vi "TreeFirstitem.vi"(8 "error in (no error)":errorcluster, 10 "queue in":refnum<queue>, 11 "TreeControl in":refnum<vi>) -> (0 "error out":errorcluster)   [LabVIEW 2019]
doc: "If the tree has values select the first and send the queue to show it"
uses:
  <vilib>/Bytelabs/ByteSimpleQ/ByteSimpleQ/Typedefs/message_cluster.ctl
  TypeDef/SubPanelType.ctl
  <vilib>/Bytelabs/ByteSimpleQ/ByteSimpleQ/ByteSimpleQ.lvlib
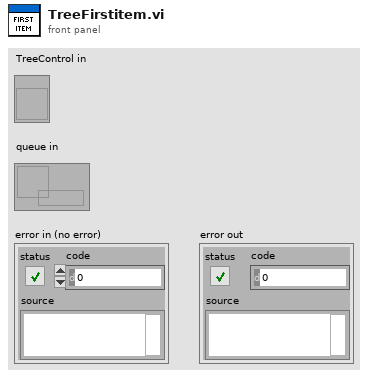
[diagram p1: front panel]
types:
  T1 = typedef "SubPanelType.ctl" = cluster{"Modality":string, "Tag":string}
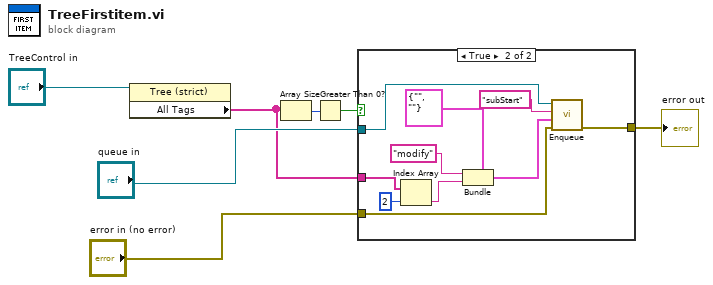
[diagram p0: block diagram]
diagram:
  n1 = property class="Tree (strict)"(reference="TreeControl in") -> ("All Tags"=w3:string[])  [unwired: 1 in, 2 out]
  n2 = Array Size(array=w3) -> (size(s)=w4:i32)
  n3 = Greater Than 0?(x=w4) -> (x > 0?=w5:bool)
  n4 = case shown="True" w5 {
    tunnel: "queue in" -> [_ w12]
    tunnel: "error in (no error)" -> [w8 w14]
    tunnel: [w8 w13] -> w1
    tunnel: w3 -> [_ w11]
    frame False {
    }
    frame True {
      n5 = Index Array(array=w11, index=2) -> (element=w9:string)
      n6 = Bundle(cluster=T1 {"Modality"="", "Tag"=""}, "Modality"="modify", "Tag"=w9) -> (w17:T1)
      n7 = call <vilib>:"Enqueue.vi"("error in (no error)"=w14, "data"=w17, "message"="subStart", "queue in"=w12) -> ("error out"=w13:errorcluster)  [unwired: 5 in, 2 out]
    }
  }
  "error out" <- w1
